vi "GLOBALS.vi"() -> ()   [LabVIEW 2019]
panel:
  in  "Tab Control":enum32{"Page 1", "Page 2"}(tab)
  in  "Valor_puro":dbl
  in  "PITOT":dbl
  in  "error in (no error)":errorcluster
  in  "TERMICO":dbl
  in  "Chaveado":dbl
  in  "Kalman_fused":dbl
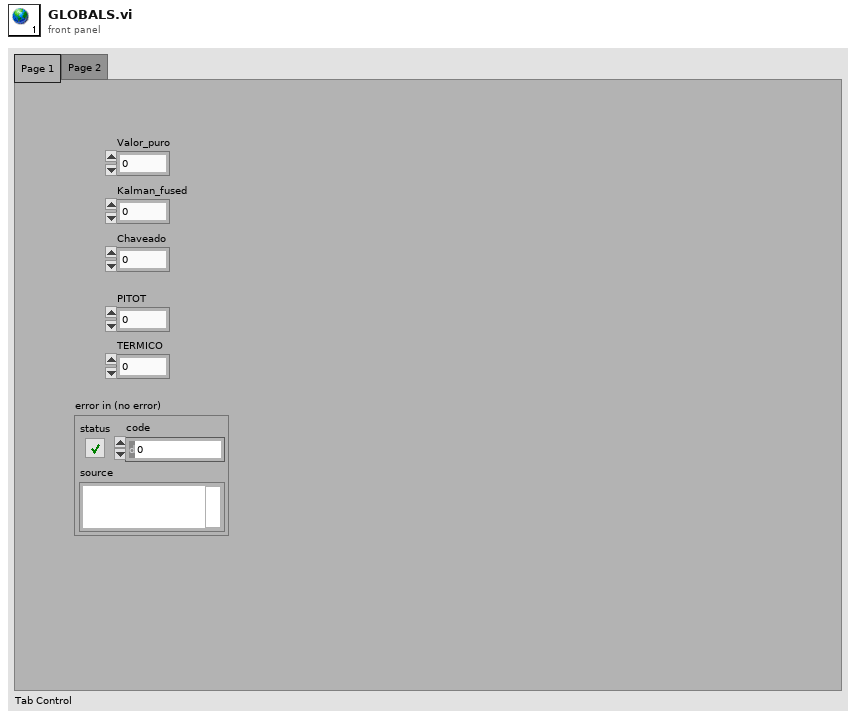
[diagram p1: front panel]
diagram:
